vi "CamDef.vi"() -> ()   [LabVIEW 2013]
panel:
  out "CamDef":bool
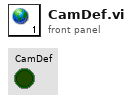
[diagram p1: front panel]
diagram:
